vi "PassBestReceiverRole.vi"(6 "Tactic index in":i32, 7 "first call":bool, 8 "error in (no error)":errorcluster, 9 "Robot":refnum<class "Robot.lvclass">, 10 "Game in":refnum<class "Game.lvclass">, 11 "PassBestReceiverRole in":refnum<class "PassBestReceiverRole.lvclass">) -> (0 "error out":errorcluster, 1 "tactic index":i32, 2 "Robot out":refnum<class "Robot.lvclass">, 3 "PassBestReceiverRole out":refnum<class "PassBestReceiverRole.lvclass">)   [LabVIEW 2024, in "PassBestReceiverRole.lvclass"]
uses:
  PassBestReceiverRole.lvclass
  C:/Users/moise/Documents/GitHub/SSL_AI/Role_class/Role.lvclass
  Robot_class/Robot.lvclass
  Game_class/Game.lvclass
  Utilities_class/Utilities.lvclass
  Role_class/Role.lvclass/Role.ctl
  Tacticbook_class/Tacticbook.lvclass/Tacticbook.ctl
  Tacticbook_class/Read WaitPassTactic.vi
  Tacticbook_class/Write WaitPassTactic.vi
  Role_class/Read Tacticbook.vi
  Role_class/Write Tacticbook.vi
  Role_class/Write tactic_index.vi
  Tacticbook_class/Tacticbook.lvclass
  WaitPassTactic_class/WaitPassTactic.lvclass
panel:
  out "Game out":refnum<class "Game.lvclass">
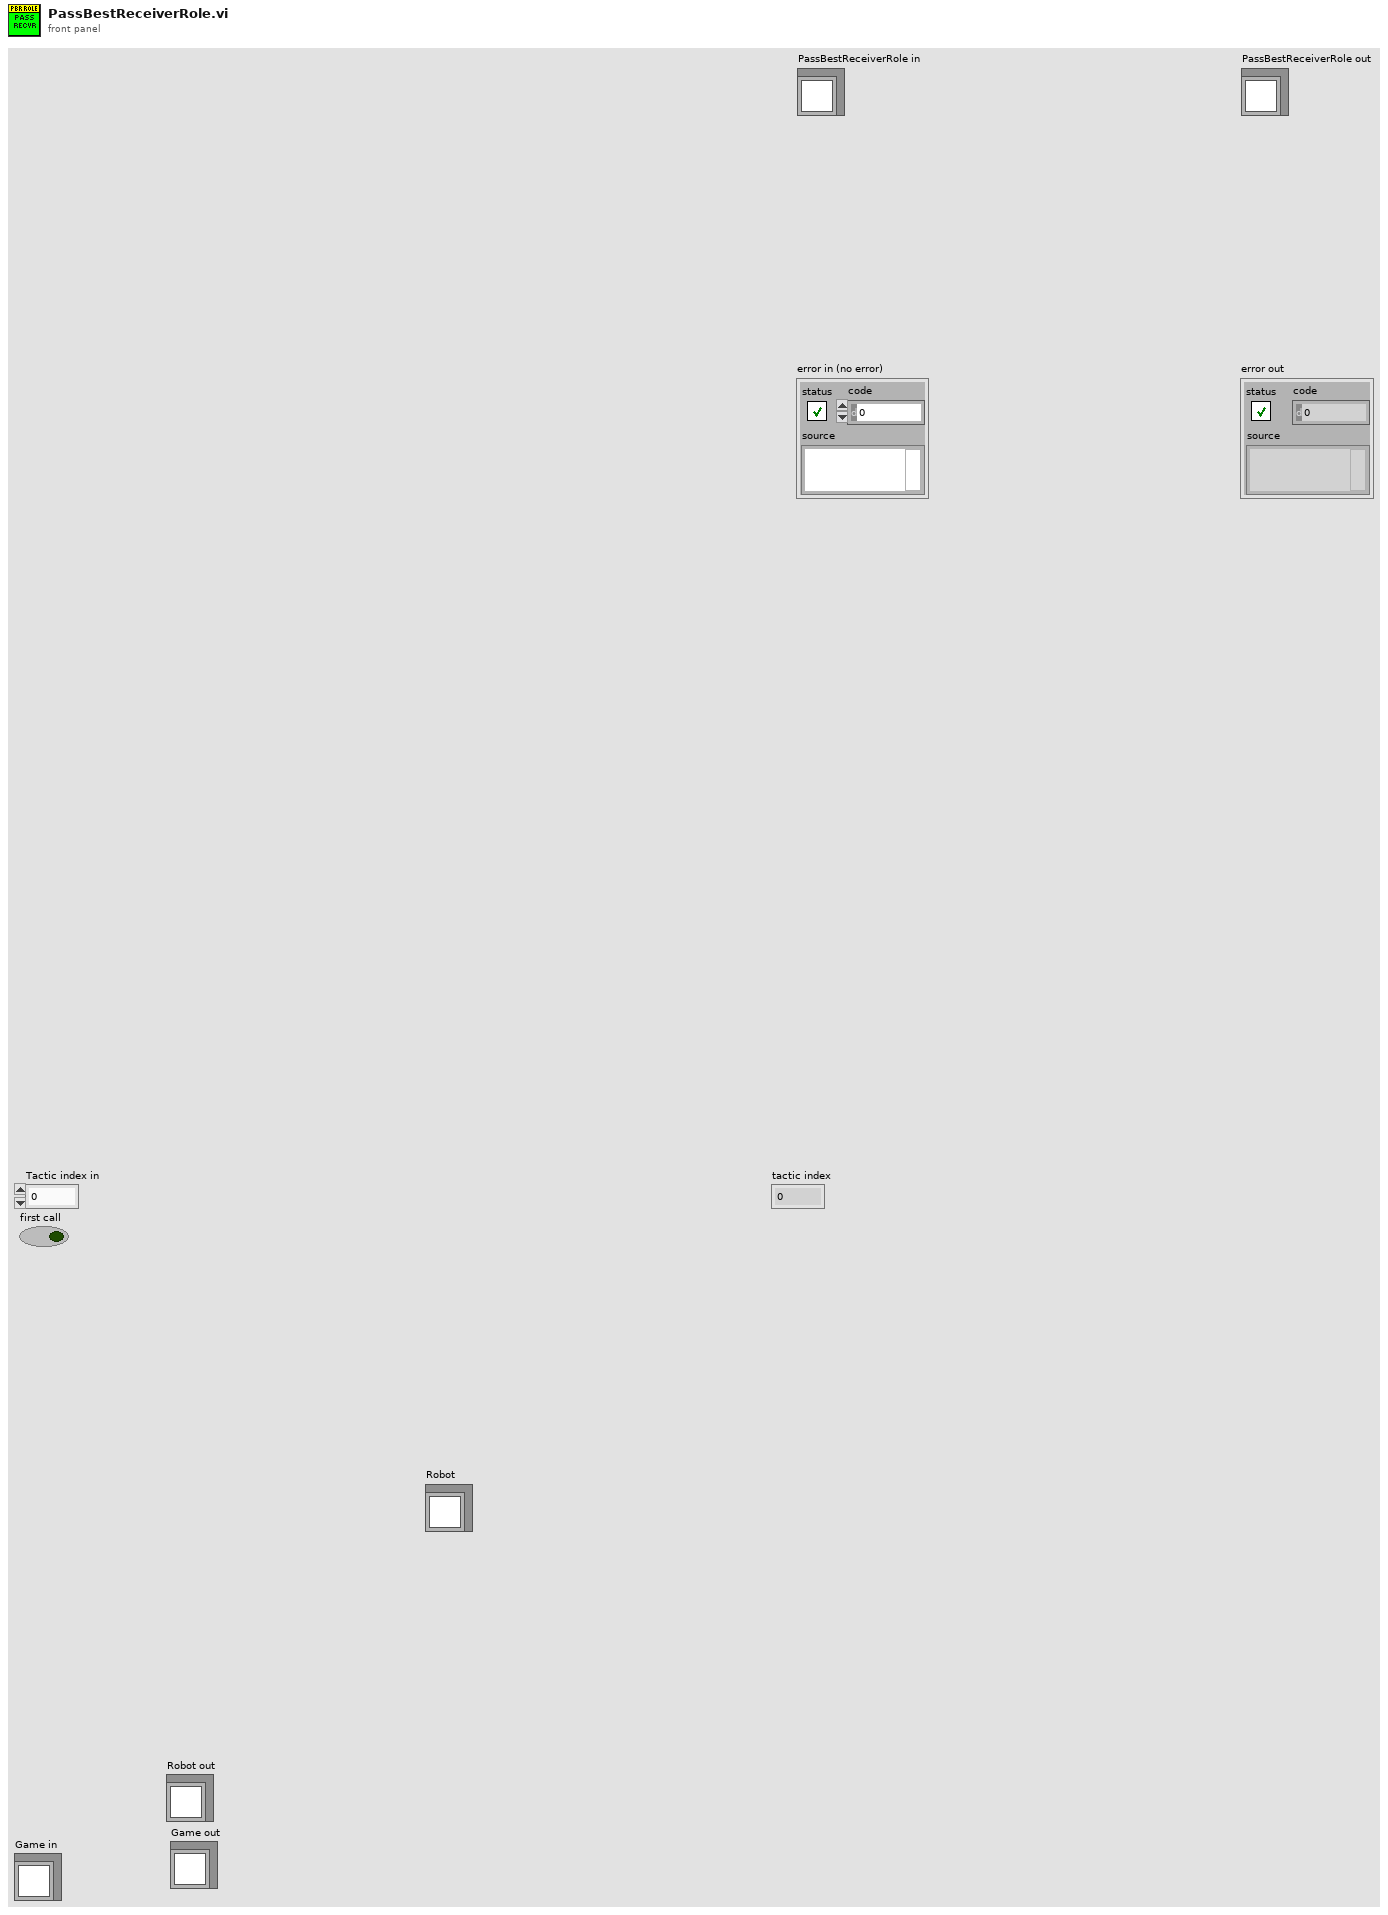
[diagram p1: front panel]
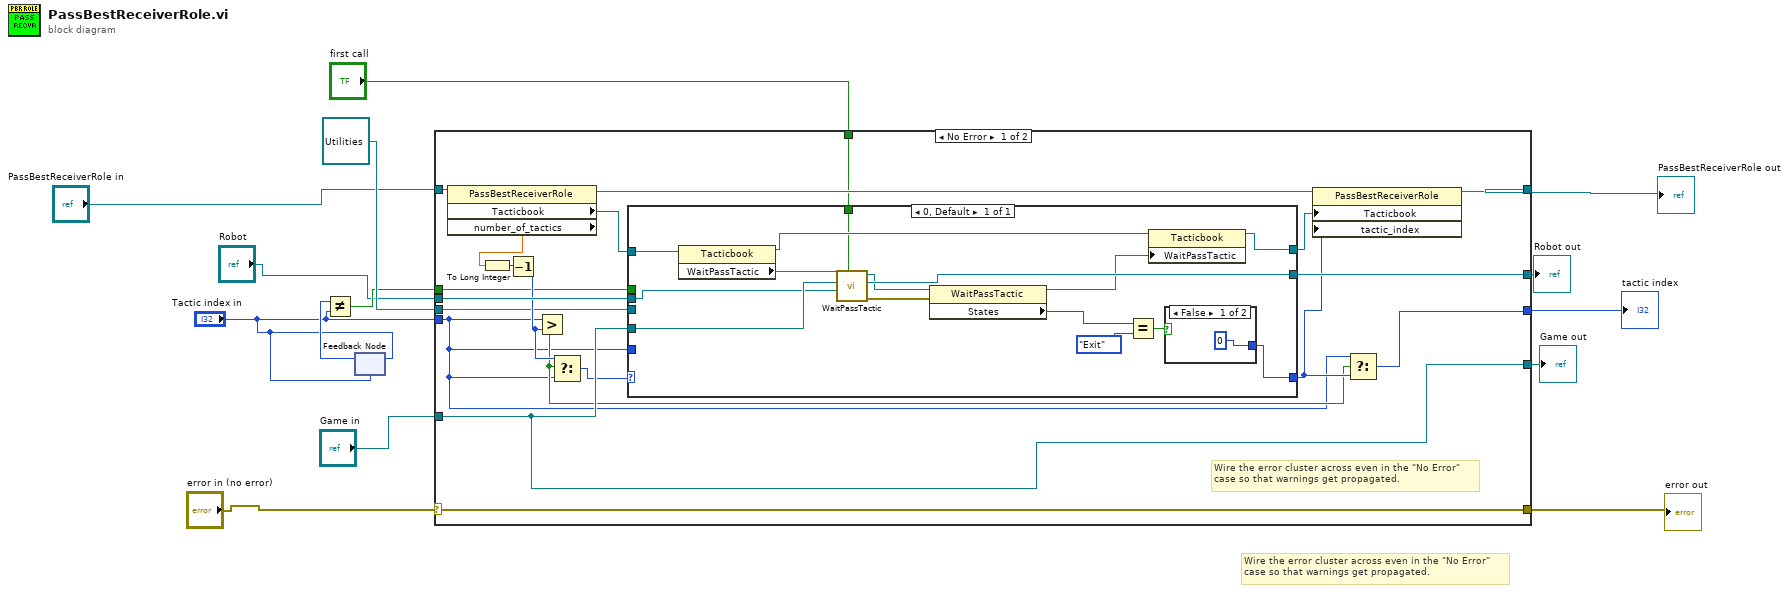
[diagram p0: block diagram]
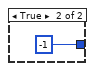
[diagram p2: hidden frame]
diagram:
  # "Wire the error cluster across even in the \"No Error\"\ncase so that warnings get propagated."
  n1 = feedback #1("Tactic index in") -> (w8:i32)
  n2 = Not Equal?(x=w8, y="Tactic index in") -> (x != y?=w6:bool)
  n3 = feedback-in #1("Tactic index in") -> ()
  n4 = case shown="No Error" "error in (no error)" {
    selector: "error in (no error)" -> [w34 w55]
    tunnel: [w34 w55] -> w4
    tunnel: [w32 w54] -> w3
    tunnel: "PassBestReceiverRole in" -> [w33 w54]
    tunnel: "Robot" -> [w29 w53]
    tunnel: [w28 w53] -> w14
    tunnel: [w26 w52] -> w13
    tunnel: "Game in" -> [w26 w52]
    tunnel: [w21 _] -> w11
    tunnel: "Tactic index in" -> [w20 _]
    tunnel: refnum<class "Utilities.lvclass"> refnum ("Utilities in") -> [w19 _]
    tunnel: "first call" -> [w18 _]
    tunnel: w6 -> [w15 _]
    frame No Error {
      # "Wire the error cluster across even in the \"No Error\"\ncase so that warnings get propagated."
      n5 = property class="PassBestReceiverRole"(reference=w33) -> (reference out=w31:refnum<class "PassBestReceiverRole.lvclass">, "Tacticbook"=w30:refnum<class "Tacticbook.lvclass">, "number_of_tactics"=w16:dbl)  [unwired: 1 in, 1 out]
      n6 = To Long Integer(number=w16) -> (32bit integer=w17:i32)
      n7 = Decrement(x=w17) -> (x-1=w25:i32)
      n8 = Greater?(x=w20, y=w25) -> (0:w22:bool)
      n9 = Select(t=w25, s=w22, f=w20) -> (s? t:f=w24:i32)
      n10 = case shown="0, Default" w24 {
        tunnel: [w37] -> w23
        tunnel: w30 -> [w49]
        tunnel: w29 -> [w40]
        tunnel: [w48] -> w28
        tunnel: [w44] -> w27
        tunnel: w26 -> [w41]
        tunnel: w20 -> [_]
        tunnel: w19 -> [_]
        tunnel: w18 -> [w35]
        tunnel: w15 -> [_]
        frame 0, Default {
          n11 = property class="Tacticbook"(reference=w49) -> (reference out=w46:refnum<class "Tacticbook.lvclass">, "WaitPassTactic"=w43:refnum<class "WaitPassTactic.lvclass">)  [unwired: 1 in, 1 out]
          n12 = call-dynamic "WaitPassTactic.vi"("first call"=w35, "Robot"=w40, "Game in"=w41, "WaitPassTactic in"=w43) -> ("error out"=w47:errorcluster, "Robot out"=w48:refnum<class "Robot.lvclass">, "WaitPassTactic out"=w42:refnum<class "WaitPassTactic.lvclass">)  [unwired: 5 in]
          n13 = property class="WaitPassTactic"(reference=w42, error in=w47) -> (reference out=w45:refnum<class "WaitPassTactic.lvclass">, "States"=w38:enum16{"State 0", "State 1", "State 2", "Exit"})  [unwired: 1 out]
          n14 = Equal?(x=w38, y=enum16{"State 0", "State 1", "State 2", "Exit"}."Exit") -> (x = y?=w39:bool)
          n15 = property class="Tacticbook"(reference=w46, "WaitPassTactic"=w45) -> (reference out=w44:refnum<class "Tacticbook.lvclass">)  [unwired: 1 in, 1 out]
          n16 = case shown="False" w39 {
            tunnel: [0 -1] -> w37
            frame False {
            }
            frame True {
            }
          }
        }
      }
      n17 = property class="PassBestReceiverRole"(reference=w31, "Tacticbook"=w27, "tactic_index"=w23) -> (reference out=w32:refnum<class "PassBestReceiverRole.lvclass">)  [unwired: 1 in, 1 out]
      n18 = Select(t=w20, s=w22, f=w23) -> (s? t:f=w21:i32)
    }
    frame Error {
    }
  }
  "error out" <- w4
  "PassBestReceiverRole out" <- w3
  "Robot out" <- w14
  "Game out" <- w13
  "tactic index" <- w11
